vi "UserVars-Permute Vector.vi"(0 "Seed":i32, 2 "Action":enum16{"Clear", "Select"}(ring)=enum."Select", 7 "N":i32, 11 "error in (no error)":errorcluster) -> (4 "Array":i32[](array[numeric]), 15 "error out":errorcluster)   [LabVIEW 2020]
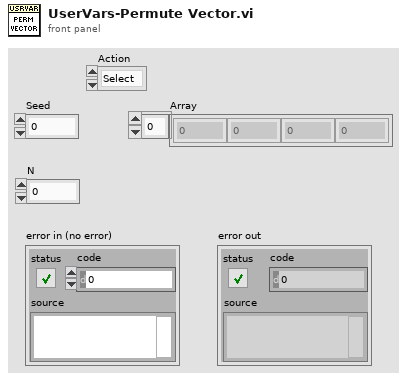
[diagram p1: front panel]
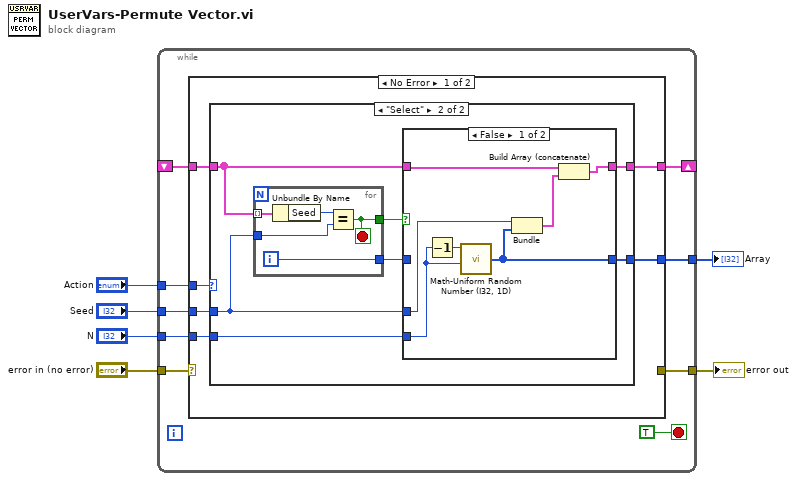
[diagram p0: block diagram]
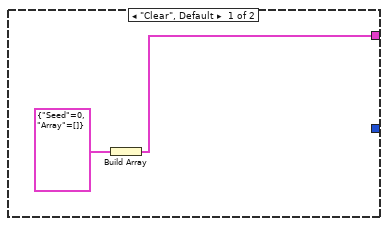
[diagram p2: hidden frame]
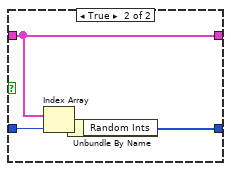
[diagram p3: hidden frame]
diagram:
  n1 = while {
    tunnel: "Action" -> [w14]
    tunnel: "Seed" -> [w13]
    tunnel: "N" -> [w12]
    shift-right: [w11] -> _
    shift-left: _ -> [w10]
    tunnel: [w9] -> w3
    tunnel: "error in (no error)" -> [w8]
    tunnel: [w7] -> w1
    stop <- TRUE stop-if-true
    n2 = case shown="No Error" w8 {
      selector: w8 -> [_ w48]
      tunnel: w14 -> [w21 _]
      tunnel: w13 -> [w20 _]
      tunnel: w12 -> [w19 _]
      tunnel: [w18 w47] -> w11
      tunnel: w10 -> [w17 w47]
      tunnel: [w16 _] -> w9
      tunnel: [_ w48] -> w7
      frame No Error {
        n3 = case shown="\"Select\"" w21 {
          tunnel: w20 -> [_ w26]
          tunnel: w19 -> [_ w25]
          tunnel: [w22 w24] -> w18
          tunnel: w17 -> [_ w29]
          tunnel: [_ w27] -> w16
          frame "Clear", Default {
            n4 = Build Array(cluster{"Seed":i32, "Array":i32[]} {"Seed"=0, "Array"=[]}) -> (w22:cluster{"Seed":i32, "Array":i32[]}[])
          }
          frame "Select" {
            n5 = for {
              tunnel: w29 -> [w46] mode=indexing
              tunnel: w26 -> [w44]
              tunnel: [w43] -> w30
              tunnel: [w42] -> w28
              i -> [w42]
              stop <- w43 stop-if-true
              n6 = Unbundle By Name(w46) -> ("Seed"=w45:i32)
              n7 = Equal?(x=w45, y=w44) -> (x = y?=w43:bool)
            }
            n8 = case shown="False" w30 {
              tunnel: w29 -> [w34 w38]
              tunnel: w28 -> [_ w41]
              tunnel: [w35 w39] -> w27
              tunnel: w26 -> [w37 _]
              tunnel: w25 -> [w36 _]
              tunnel: [w32 w38] -> w24
              frame False {
                n9 = Decrement(x=w36) -> (x-1=w31:i32)
                n10 = call "Math-Uniform Random Number (I32, 1D).vi"("N"=w36, "Ymax"=w31) -> ("Random Ints"=w35:i32[])  [unwired: 4 in]
                n11 = Bundle("Seed"=w37, "Random Ints"=w35) -> (w33:cluster{"Seed":i32, "Random Ints":i32[]})  [unwired: 1 in]
                n12 = Build Array (concatenate)(w34, w33) -> (w32:cluster{"Seed":i32, "Random Ints":i32[]}[])
              }
              frame True {
                n13 = Index Array(array=w38, index=w41) -> (element=w40:cluster{"Seed":i32, "Random Ints":i32[]})
                n14 = Unbundle By Name(w40) -> ("Random Ints"=w39:i32[])
              }
            }
          }
        }
      }
      frame Error {
      }
    }
  }
  "Array" <- w3
  "error out" <- w1
